vi "MGCC_visualization_phasetwo.vi"() -> ()   [LabVIEW 2016]
panel:
  in  "TEST CASE":string(combo)
  out "SM_G1L3L6L7":bool
  out "SM_G1L3L6":bool
  out "LI_L5_SW_L5L3_2":bool
  out "LI_L5_SW_L5L3_1":bool
  out "SM_L2L3L5":bool
  out "LI_SW_G1L3_L3_4":bool
  out "LI_SW_G1L3_L3_3":bool
  out "B2":bool
  out "SOC Tank 2":dbl(slide) scale=0.0..1.0
  out "LI_SW_L3L6_L6_1":bool
  out "PV1":bool
  out "B1":bool
  out "LI_SW_G1L3_L3_2":bool
  out "LI_L3_SW_L3L4":bool
  out "LI_L1_SW_L1L3_2":bool
  out "SOC Tank":dbl(slide) scale=0.0..1.0
  out "L2":bool
  out "LI_SW_L3L2_L2_2":bool
  out "LI_L2_B2_2":bool
  out "LI_SW_L6L7_L7_1":bool
  out "SW_L6_L7":bool
  out "L1":bool
  out "L6":bool
  out "LI_L6_SW_L6L7":bool
  out "LI_SW_L3L6_L6_2":bool
  out "SW_L3_L6":bool
  out "SW_L3_L4":bool
  out "SW_L3_L2":bool
  out "LI_G1_SW_G1L3":bool
  out "SW_G1L3":bool
  out "G1":bool
  out "LI_B_SW_L1L3_2":bool
  out "LI_SW_L1L3_L3":bool
  out "SW_L1_L3":bool
  out "L5":bool
  out "SW_L5_L3":bool
  out "L7":bool
  out "LI_SW_L6L7_L7_2":bool
  out "LI_L2_B2_1":bool
  out "LI_SW_L3L4_L4_1":bool
  out "L4":bool
  out "LI_SW_L3L4_L4_2":bool
  out "L3":bool
  out "PV1 irr Tank":dbl(slide) scale=0.0..10.0
  out "LI_L3_SW_L3L2":bool
  out "LI_SW_L5L3_L3":bool
  out "LI_L3_SW_L3L6":bool
  out "LI_SW_G1L3_L3_1":bool
  out "LI_SW_L3L2_L2_1":bool
  out "LI_B_SW_L1L3":bool
  out "LI_L1_SW_L1L3_1":bool
  out "LI_PV_SW_L1L3":bool
  out "SM_L1L3":bool
  out "SM_L1":bool
  out "SM_L1L3L5":bool
  out "SM_G1L1L3L5":bool
  out "SM_L2L4L5L6L7":bool
  out "SM_L2L3L4":bool
  out "SM_L1L3L4":bool
  out "SM_all":bool
  out "SM_L2":bool
  # "G1"
  # "SW2"
  # "SW1"
  # "SW3"
  # "L6"
  # "L7"
  # "SW4"
  # "SW5"
  # "L5"
  # "L2"
  # "BESS2"
  # "SW7"
  # "SW6"
  # "L3"
  # "L4"
  # "L1"
  # "BESS1"
  # "PV1"
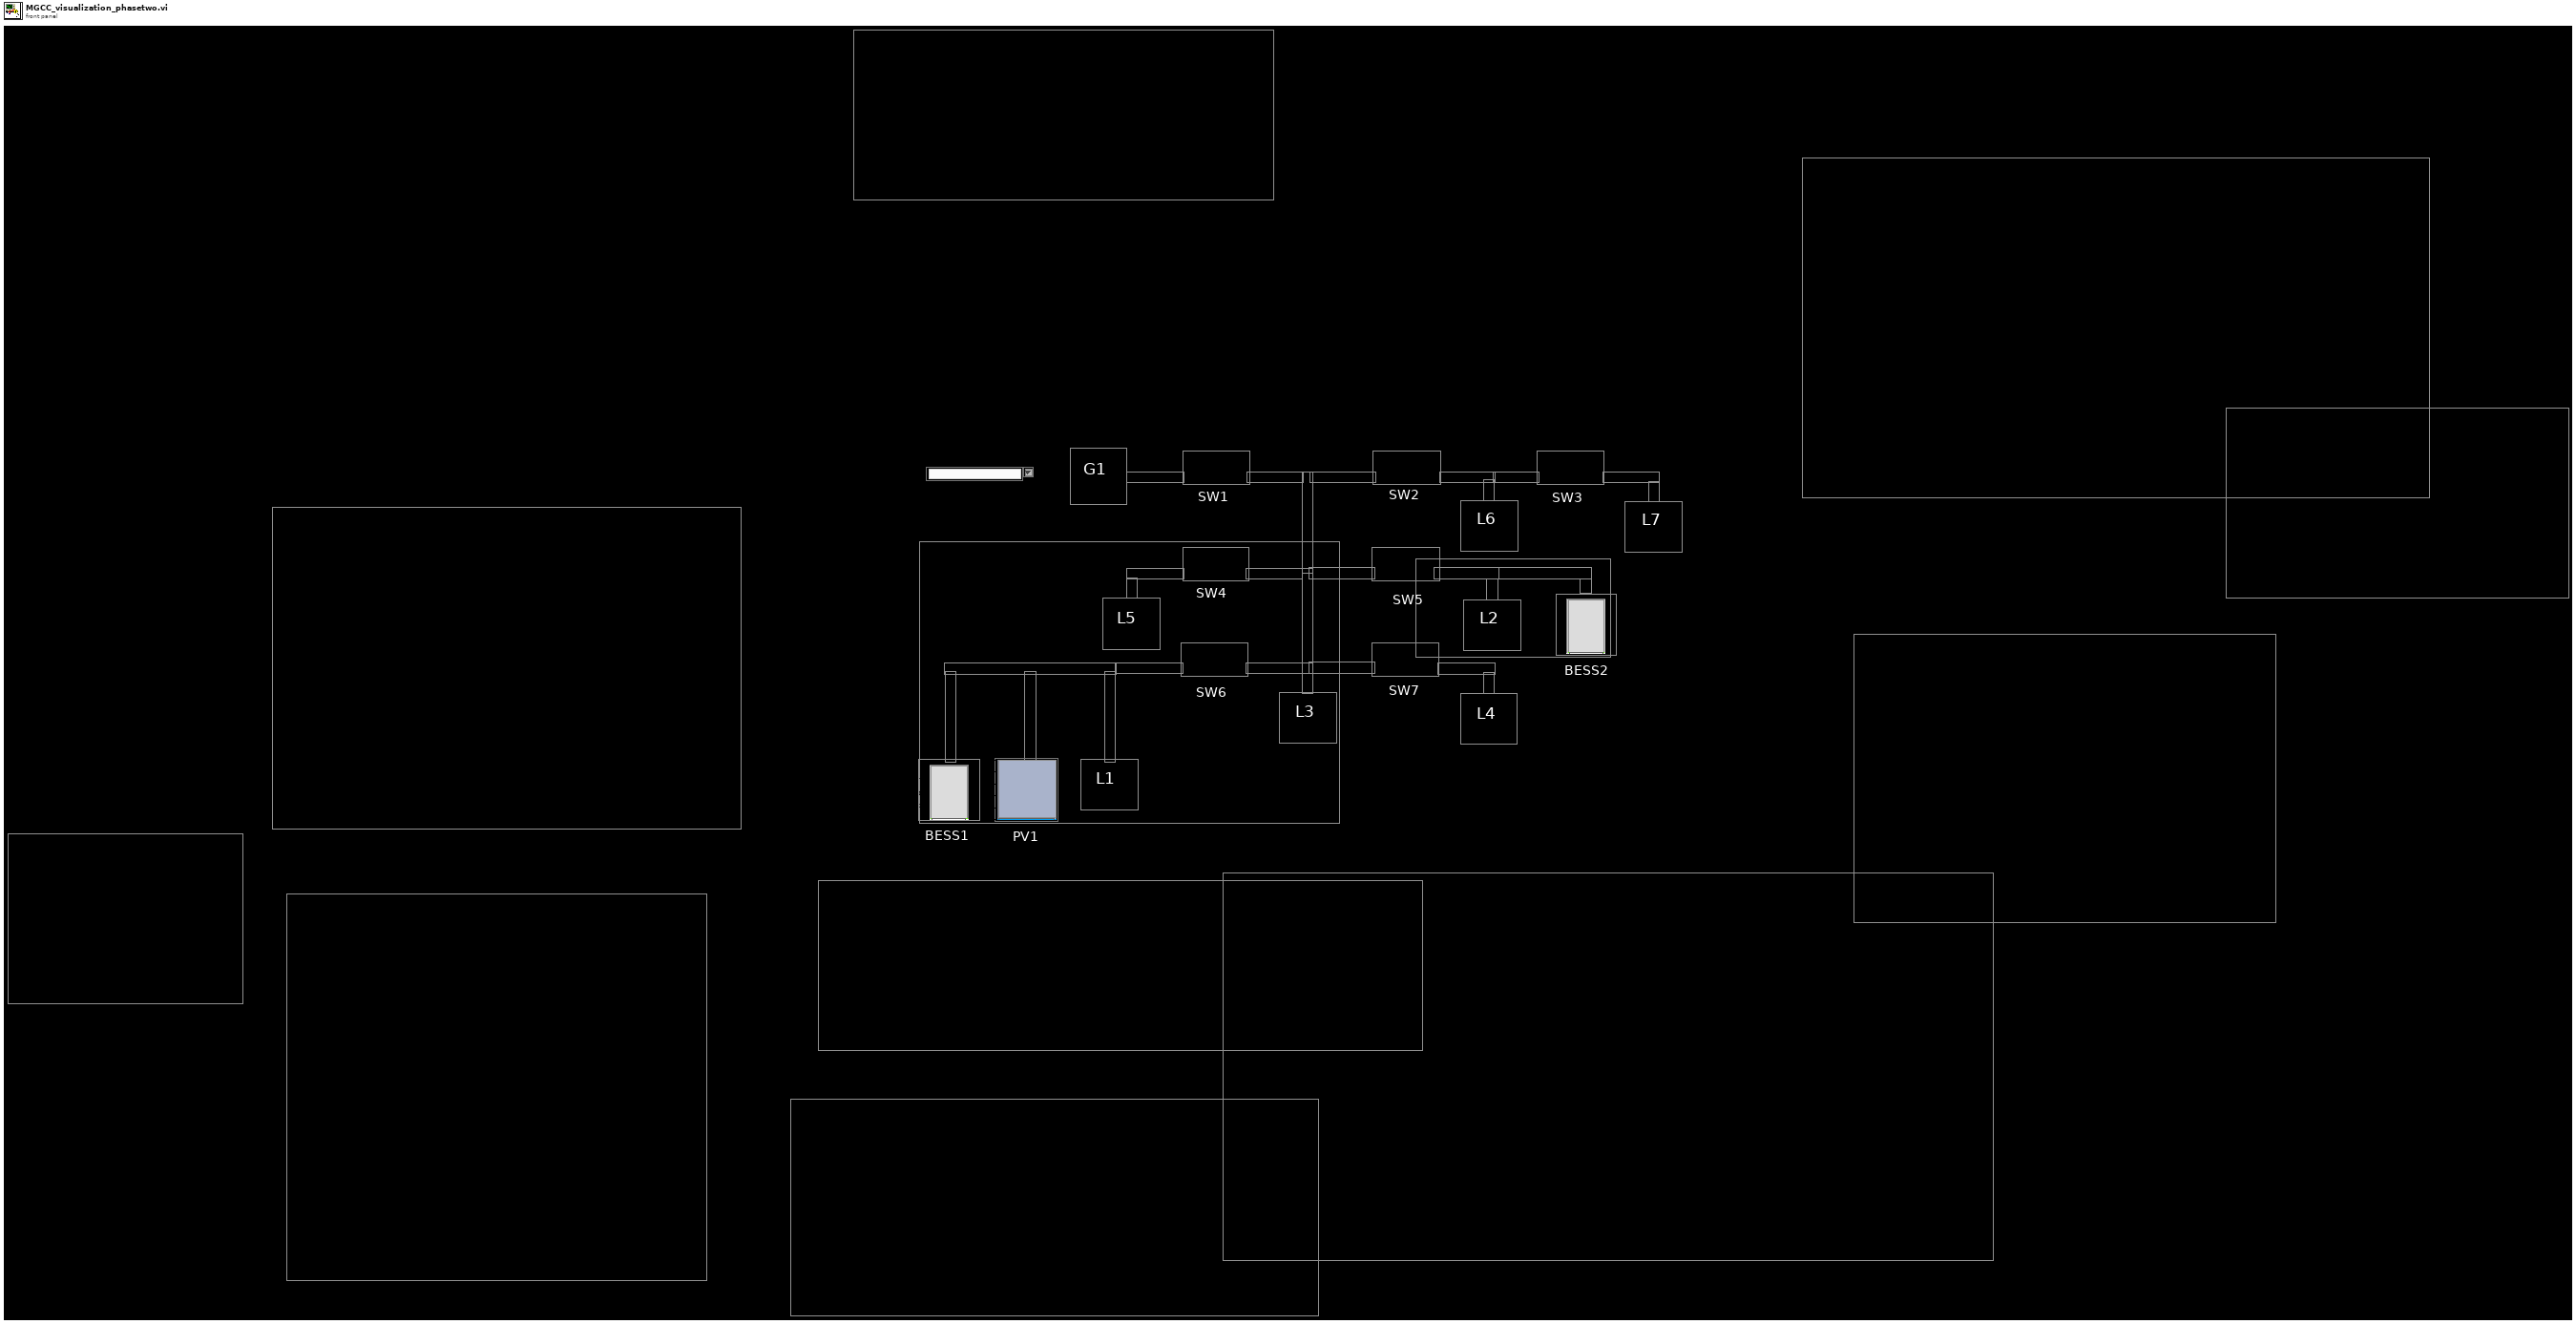
[diagram p1: front panel]
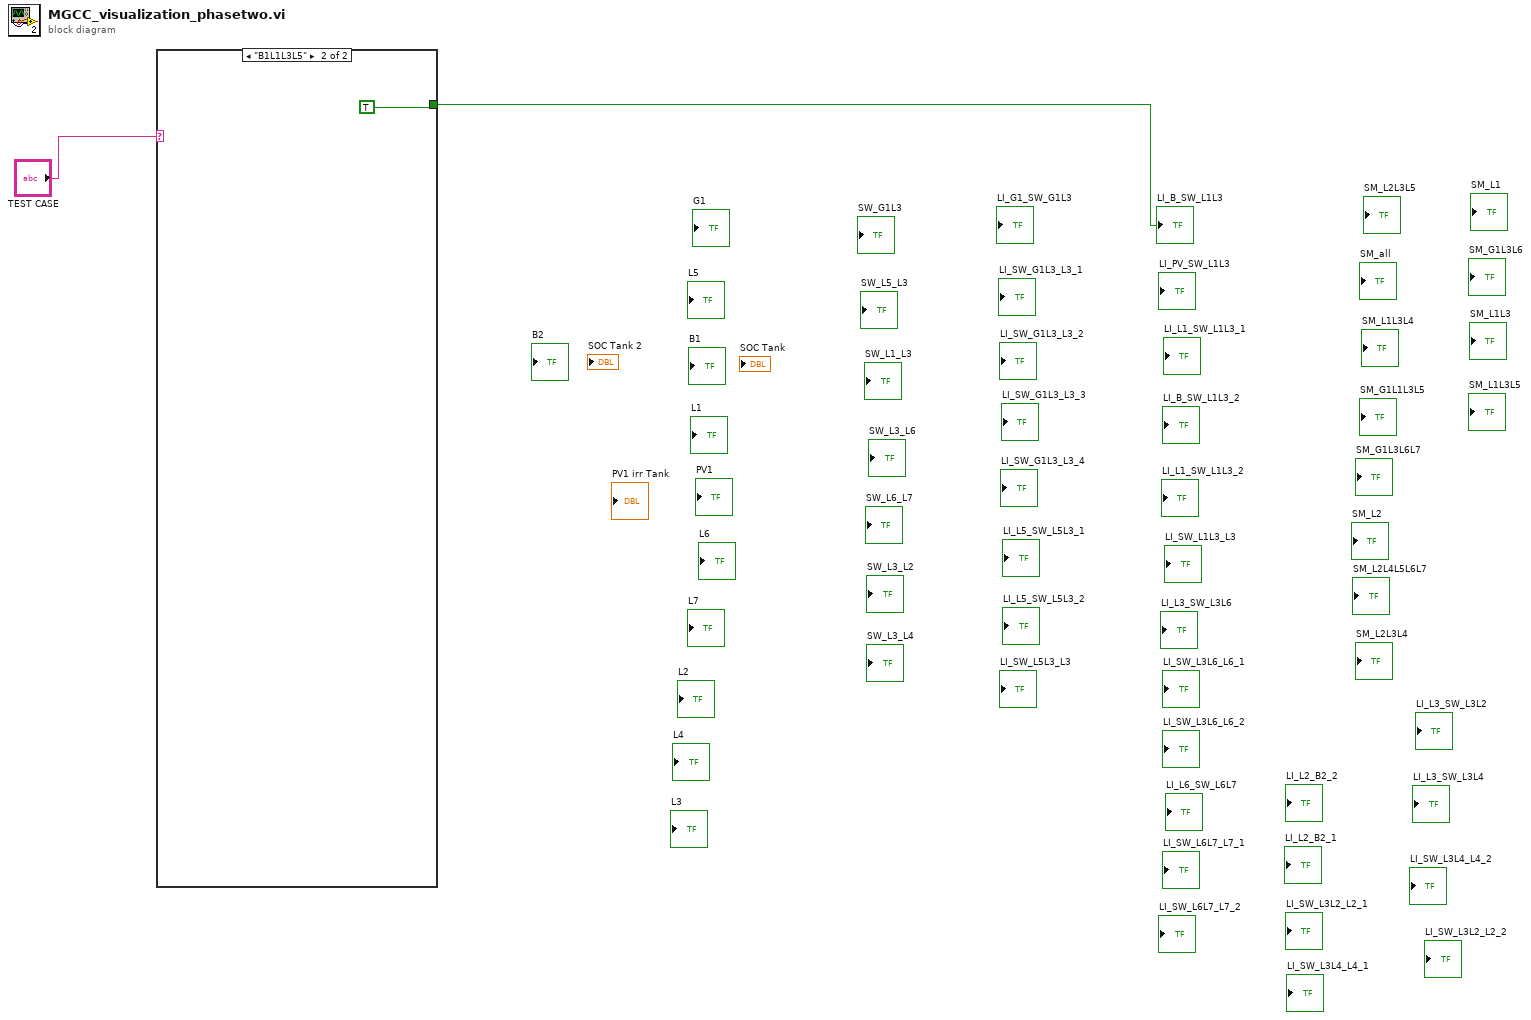
[diagram p0: block diagram]
diagram:
  n1 = case shown="\"B1L1L3L5\"" "TEST CASE" {
    tunnel: [_ TRUE] -> w1
    frame "B1L1L3L5&B2L2" {
    }
    frame "B1L1L3L5" {
    }
  }
  "LI_B_SW_L1L3" <- w1
